vi "Merge Error.vi"(10 "Error":errorcluster, 11 "Dev Actor in":refnum<class "Dev Actor.lvclass">) -> (3 "Dev Actor out":refnum<class "Dev Actor.lvclass">)   [LabVIEW 2021, in "Dev Actor.lvlib" / "Dev Actor.lvclass"]
uses:
  Dev Actor.lvclass
  Dev Actor.lvclass/Dev Actor.ctl
  Actor/Queue Actor/Queue Actor.lvclass
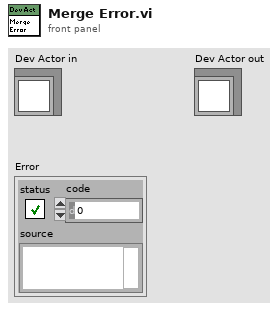
[diagram p1: front panel]
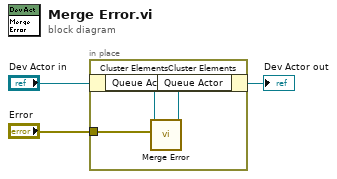
[diagram p0: block diagram]
diagram:
  n1 = in-place {
    in-place-border: "Error" -> [w5]
    n2 = in-place-cluster #1("Dev Actor in") -> ("Queue Actor"=w6:refnum<class "Queue Actor.lvclass">)
    n3 = call-dynamic "Merge Error.vi"("Error"=w5, "Set Error in"=w6) -> ("Set Error out"=w4:refnum<class "Queue Actor.lvclass">)  [unwired: 9 in]
    n4 = in-place-cluster #1("Queue Actor"=w4) -> (→"Dev Actor out":refnum<class "Dev Actor.lvclass">)
  }
